vi "TestTMflexDatabase1.vi"() -> ()   [LabVIEW 2014]
uses:
  TMflexDatabase.lvclass
  <vilib>/Utility/config.llb/Read Key (String).vi
  <vilib>/Utility/config.llb/Write Key (String).vi
  <vilib>/Utility/config.llb/NI_LVConfig.lvlib
panel:
  out "ConnectionString":string
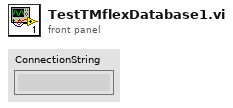
[diagram p1: front panel]
types:
  T1 = typedef "NI_LVConfig.lvlib/Config Data RefNum.ctl" = refnum<k1>
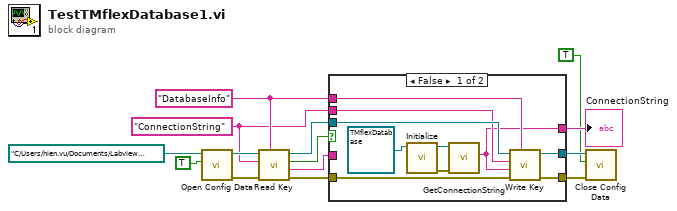
[diagram p0: block diagram]
diagram:
  w5 = "DatabaseInfo" ("section")
  w4 = "ConnectionString" ("key")
  n1 = call <vilib>:"Open Config Data.vi"("create file if necessary (T)"=TRUE, "configuration file path"=path "C:/Users/hien.vu/Documents/Labview Exercise/TMflexDatabase/TestTMflexDatabase.ini") -> ("error out"=w11:errorcluster, "refnum"=w12:T1)  [unwired: 7 in, 1 out]
  n2 = call-poly <vilib>:"Read Key.vi"("section"=w5, "error in (no error)"=w11, "key"=w4, "refnum"=w12) -> ("error out"=w6:errorcluster, "value"=w9:string, "found?"=w10:bool, "refnum out"=w7:T1)  [unwired: 4 in]
  n3 = case shown="False" w10 {
    tunnel: [w17 w27] -> w8
    tunnel: w9 -> [_ w27]
    tunnel: w7 -> [w24 w25]
    tunnel: w6 -> [w23 w26]
    tunnel: w5 -> [w22 _]
    tunnel: w4 -> [w21 _]
    tunnel: [w15 w26] -> w3
    tunnel: [w16 w25] -> w2
    frame False {
      n4 = call-dynamic "Initialize.vi"("TMflexDatabase in"=refnum<class "TMflexDatabase.lvclass"> refnum ("TMflexDatabase.lvclass")) -> ("error out"=w18:errorcluster, "TMflexDatabase out"=w19:refnum<class "TMflexDatabase.lvclass">)  [unwired: 9 in]
      n5 = call-dynamic "GetConnectionString.vi"("error in (no error)"=w18, "TMflexDatabase in"=w19) -> ("ConnectionString"=w17:string)  [unwired: 7 in, 2 out]
      n6 = call-poly <vilib>:"Write Key.vi"("section"=w22, "error in (no error)"=w23, "value"=w17, "key"=w21, "refnum"=w24) -> ("error out"=w15:errorcluster, "refnum out"=w16:T1)  [unwired: 4 in, 1 out]
    }
    frame True {
    }
  }
  "ConnectionString" <- w8
  n7 = call <vilib>:"Close Config Data.vi"("error in (no error)"=w3, "write file if changed (T)"=TRUE, "refnum"=w2) -> ()  [unwired: 7 in, 2 out]
